vi "genHelpFileOut.vi"(0 "Output Cluster":T1) -> (5 "Help Description":string="Simulated Analog Input\nNumber of Samples: 100.000000\nSampling Frequency (Hz): 1000.000000\nNumber of Channels: 2.000000\nNumber of Samples 2: 10.000000\nSampling Frequency2 (Hz): 100.000000\nNumber of Channels 2: 0.000000")   [LabVIEW 2020]
uses:
  <vilib>/express/express shared/propPageData.ctl
panel:
  in  "File Path":string="File Path:"
  in  "Lock File":string="Lock File:"
  in  "Lock File enum":string[](array[string])=[" False", " True"]
  in  "Delimiter enum":string[](array[string])=["Tabulator", "Comma", "No headers"]
  in  "Delimiter":string="Delimiter:"
  in  "Segment headers enum":string[](array[string])=["One header per segment", "One header only", "No headers"]
  in  "Segment file":string="Segment headers:"
  in  "X value column enum":string[](array[string])=["Empty time column", "One column only", "One column per channel"]
  in  "X value column":string="X value(time) columns: "
  in  "Format enum":string[](array[string])=["Text (LVM)", "Binary with XML Header (TDM)", "Binary (TDMS)", "Microsoft Excel (.xlsx)"]
  in  "Format":string="File Format: "
  in  "File_dialog enum":string[](array[string])=[" False", " True"]
  in  "Ask user to choose file":string="Ask user to choose file:"
  in  "Multi-file or one":string[](array[string])=["Save to one file", "Save to a series of files (Multi-file)"]
  in  "Description:":string="Description: "
  in  "If a file already exists:":string="If a file already exists: "
  in  "OverWrite_mode":string[](array[string])=["Overwrite file", "Rename existing file", "Append to file", "Use next available filename "]
  in  "Mode":string="Mode: "
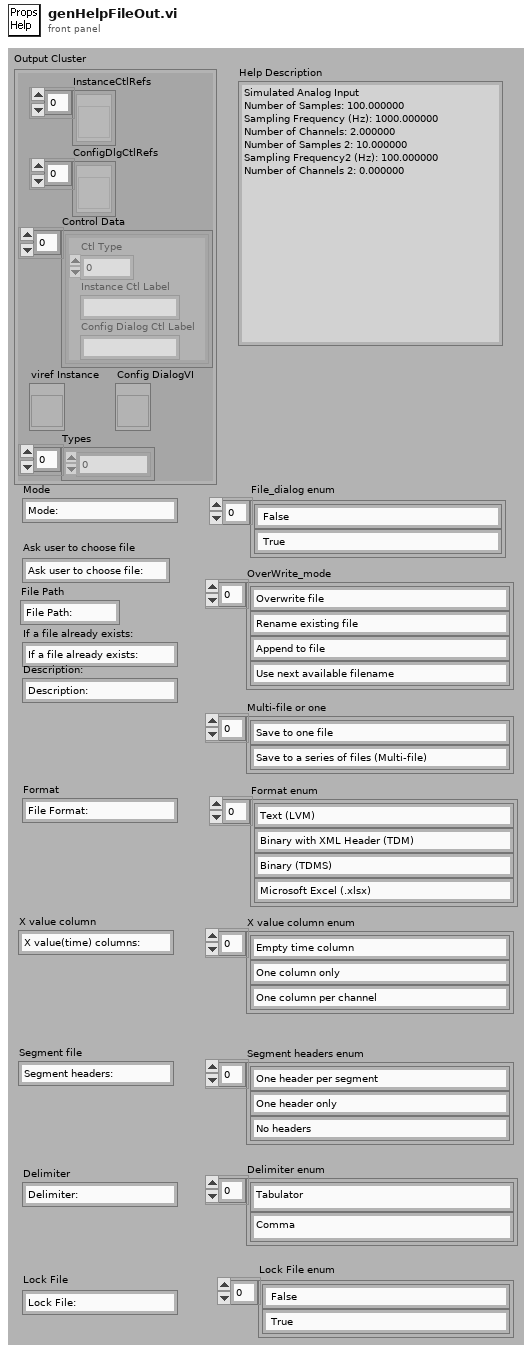
[diagram p1: front panel]
types:
  T1 = typedef "propPageData.ctl" = cluster{"InstanceCtlRefs":refnum<vi>[], "ConfigDlgCtlRefs":refnum<vi>[], "Control Data":cluster{"Ctl Type":u16, "Instance Ctl Label":string, "Config Dialog Ctl Label":string}[], "viref Instance":refnum<vi>, "Types":i32[], "Config DialogVI":refnum<vi>}
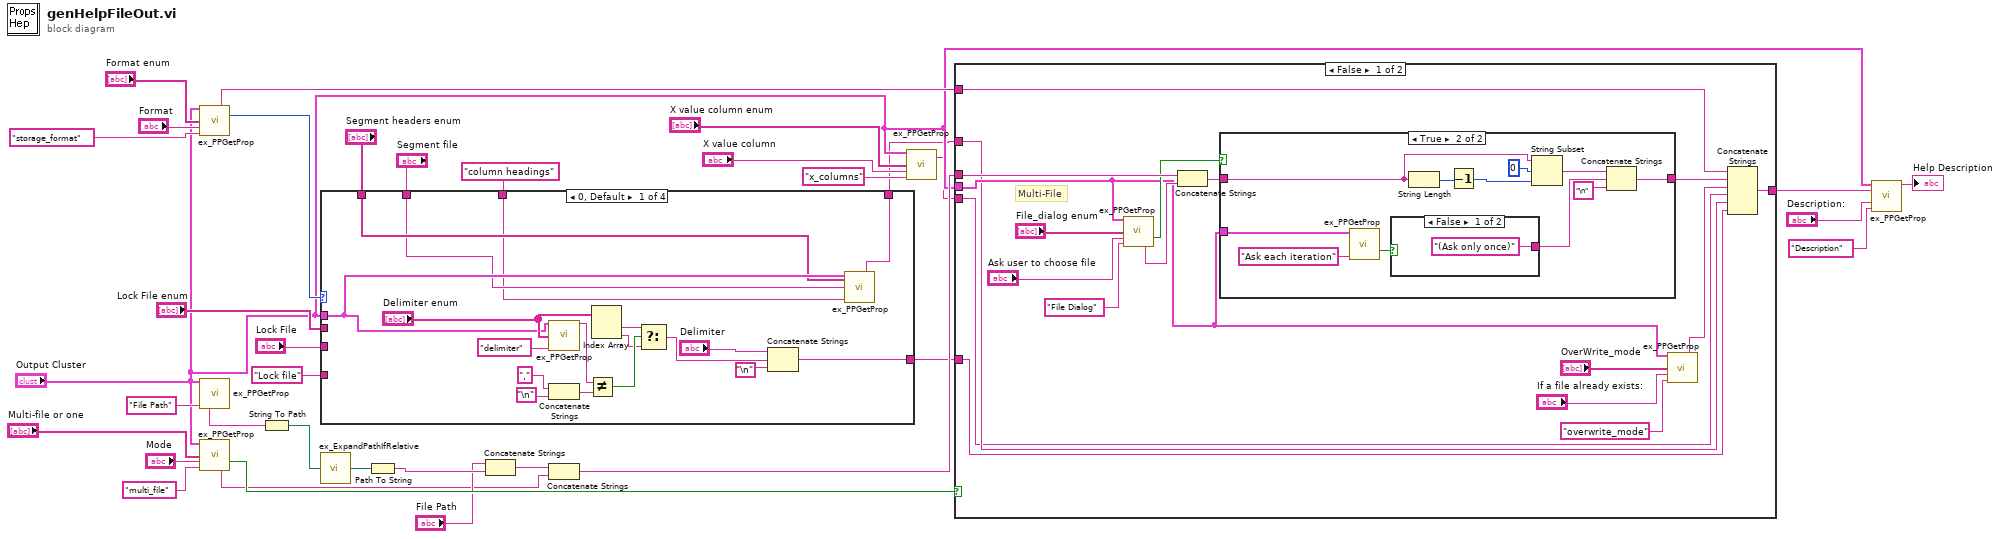
[diagram p0: block diagram]
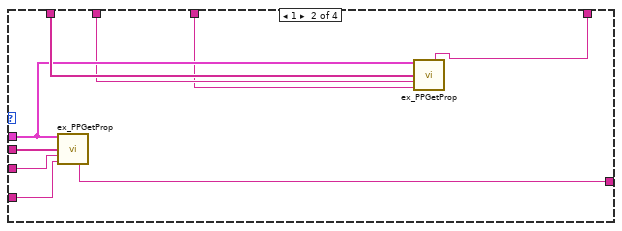
[diagram p2: hidden frame]
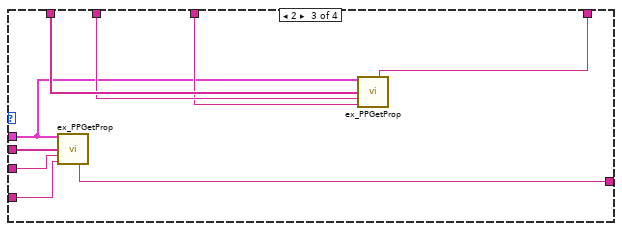
[diagram p3: hidden frame]
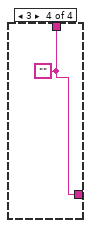
[diagram p4: hidden frame]
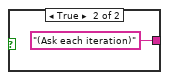
[diagram p6: hidden frame]
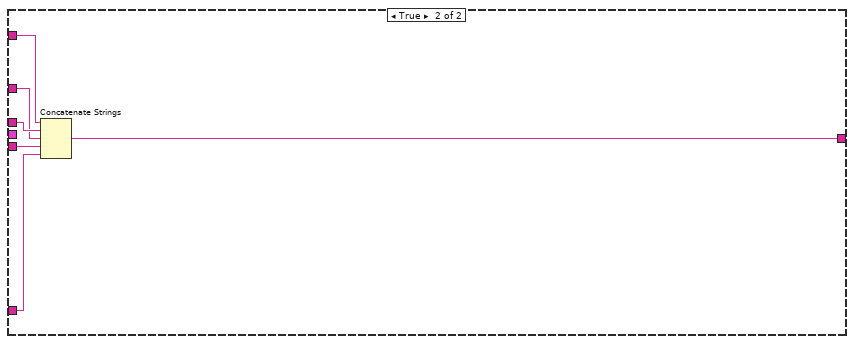
[diagram p7: hidden frame]
diagram:
  n1 = call <vilib>:"ex_PPGetProp.vi"("Output Cluster"="Output Cluster", "Enum & T/F Strings"="Format enum", "Prefix"="Format", "Control:"="storage_format") -> ("Enum Result"=w16:string, "int32"=w17:i32)  [unwired: 3 in, 7 out]
  n2 = call <vilib>:"ex_PPGetProp.vi"("Output Cluster"="Output Cluster", "Control:"="File Path") -> ("String (Path)"=w23:string)  [unwired: 5 in, 8 out]
  n3 = call <vilib>:"ex_PPGetProp.vi"("Output Cluster"="Output Cluster", "Enum & T/F Strings"="Multi-file or one", "Prefix"="Mode", "Control:"="multi_file") -> ("bool"=w27:bool, "T/F Result"=w11:string)  [unwired: 3 in, 7 out]
  n4 = String To Path(string=w23) -> (path=w22:path)
  n5 = case shown="0, Default" w17 {
    tunnel: "Output Cluster" -> [w40 w57 w64 _]
    tunnel: [w41 w60 w69 w72] -> w15
    tunnel: "Lock File enum" -> [_ w59 w68 _]
    tunnel: "Lock File" -> [_ w62 w71 _]
    tunnel: "Lock file" -> [_ w61 w70 _]
    tunnel: [w36 w54 w63 w72] -> w4
    tunnel: "Segment headers enum" -> [w39 w58 w67 _]
    tunnel: "Segment file" -> [w38 w56 w66 _]
    tunnel: "column headings" ("Control:") -> [w37 w55 w65 _]
    frame 0, Default {
      n6 = call <vilib>:"ex_PPGetProp.vi"("Output Cluster"=w40, "Enum & T/F Strings"="Delimiter enum", "Control:"="delimiter") -> ("String"=w52:string)  [unwired: 4 in, 8 out]
      n7 = Concatenate Strings("," ("y"), "\n") -> (w51:string)
      n8 = Not Equal?(x=w52, y=w51) -> (x != y?=w45:bool)
      n9 = Index Array(array="Delimiter enum") -> (element #1=w44:string, element #2=w43:string)  [unwired: 2 in]
      n10 = Select(t=w44, s=w45, f=w43) -> (s? t:f=w47:string)
      n11 = Concatenate Strings("Delimiter", w47, "\n") -> (w41:string)
      n12 = call <vilib>:"ex_PPGetProp.vi"("Output Cluster"=w40, "Enum & T/F Strings"=w39, "Prefix"=w38, "Control:"=w37) -> ("Enum Result"=w36:string)  [unwired: 3 in, 8 out]
    }
    frame 1 {
      n13 = call <vilib>:"ex_PPGetProp.vi"("Output Cluster"=w57, "Enum & T/F Strings"=w59, "Prefix"=w62, "Control:"=w61) -> ("T/F Result"=w60:string)  [unwired: 3 in, 8 out]
      n14 = call <vilib>:"ex_PPGetProp.vi"("Output Cluster"=w57, "Enum & T/F Strings"=w58, "Prefix"=w56, "Control:"=w55) -> ("Enum Result"=w54:string)  [unwired: 3 in, 8 out]
    }
    frame 2 {
      n15 = call <vilib>:"ex_PPGetProp.vi"("Output Cluster"=w64, "Enum & T/F Strings"=w68, "Prefix"=w71, "Control:"=w70) -> ("T/F Result"=w69:string)  [unwired: 3 in, 8 out]
      n16 = call <vilib>:"ex_PPGetProp.vi"("Output Cluster"=w64, "Enum & T/F Strings"=w67, "Prefix"=w66, "Control:"=w65) -> ("Enum Result"=w63:string)  [unwired: 3 in, 8 out]
    }
    frame 3 {
      w72 = ""
    }
  }
  n17 = call <vilib>:"ex_ExpandPathIfRelative.vi"("Path"=w22) -> ("Expanded path"=w21:path)  [unwired: 3 in, 1 out]
  n18 = Path To String(path=w21) -> (string=w25:string)
  n19 = Concatenate Strings("File Path", w25) -> (w10:string)
  n20 = Concatenate Strings(w10, w11) -> (w26:string)
  n21 = call <vilib>:"ex_PPGetProp.vi"("Output Cluster"="Output Cluster", "Enum & T/F Strings"="X value column enum", "Prefix"="X value column", "Control:"="x_columns") -> ("Enum Result"=w5:string)  [unwired: 3 in, 8 out]
  n22 = case shown="False" w27 {
    tunnel: w26 -> [w86 w110]
    tunnel: "Output Cluster" -> [w77 _]
    tunnel: [w80 w108] -> w31
    tunnel: w16 -> [w76 w109]
    tunnel: w15 -> [w75 w105]
    tunnel: w4 -> [w74 w107]
    tunnel: w5 -> [w73 w106]
    frame False {
      # "Multi-File"
      n23 = call <vilib>:"ex_PPGetProp.vi"("Output Cluster"=w77, "Enum & T/F Strings"="File_dialog enum", "Prefix"="Ask user to choose file", "Control:"="File Dialog") -> ("bool"=w84:bool, "T/F Result"=w85:string)  [unwired: 3 in, 7 out]
      n24 = Concatenate Strings(w86, w85) -> (w83:string)
      n25 = case shown="True" w84 {
        tunnel: w83 -> [w91 w95]
        tunnel: [w91 w100] -> w81
        tunnel: w77 -> [_ w102]
        frame False {
        }
        frame True {
          n26 = call <vilib>:"ex_PPGetProp.vi"("Output Cluster"=w102, "Control:"="Ask each iteration") -> ("bool"=w99:bool)  [unwired: 5 in, 8 out]
          n27 = case shown="False" w99 {
            tunnel: ["(Ask only once)" ("Control:") "(Ask each iteration)" ("Control:")] -> w98
            frame False {
            }
            frame True {
            }
          }
          n28 = String Length(string=w95) -> (length=w93:i32)
          n29 = Decrement(x=w93) -> (x-1=w94:i32)
          n30 = String Subset(string=w95, offset (0)=0, length (rest)=w94) -> (substring=w92:string)
          n31 = Concatenate Strings(w92, w98, "\n" ("string")) -> (w100:string)
        }
      }
      n32 = call <vilib>:"ex_PPGetProp.vi"("Output Cluster"=w77, "Enum & T/F Strings"="OverWrite_mode", "Prefix"="If a file already exists:", "Control:"="overwrite_mode") -> ("Enum Result"=w78:string)  [unwired: 3 in, 8 out]
      n33 = Concatenate Strings(w76, w81, w78, w73, w74, w75) -> (w80:string)
    }
    frame True {
      n34 = Concatenate Strings(w109, w110, w107, w106, w105) -> (w108:string)
    }
  }
  n35 = call <vilib>:"ex_PPGetProp.vi"("Output Cluster"="Output Cluster", "Previous String"=w31, "Prefix"="Description:", "Control:"="Description") -> ("String"=→"Help Description":string)  [unwired: 3 in, 8 out]
